vi "Drive Playback.vi"() -> ()   [LabVIEW 2010]
uses:
  <vilib>/NXT/Subs/MotorXNode.DC Motor Type.ctl
  <vilib>/NXT/Subs/LVHSConnector.ctl
  <vilib>/NXT/NXTIO Xnodes/NXTIOXNode/NXTIO.xnode
  <vilib>/NXT/Subs/MotorXNode.2DCMotor.ctl
  <vilib>/NXT/NXTIO Xnodes/AddressXNode/NXTIOAddress.xnode
  4150_RingItUp_State/4150_RingItUp_State.lvrbt
  <vilib>/NXT/NXTIO Xnodes/NXTIONodeSubVIs/TETRIX IO Move DC Motors.vi
panel:
  in  "DriveData":i8[][](array[numeric])
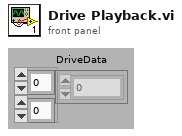
[diagram p1: front panel]
types:
  T1 = typedef "MotorXNode.DC Motor Type.ctl" = enum16{"DC Motor"}
  T2 = cluster{"DC Motor":T1, "Address":i16, "Address":i16}
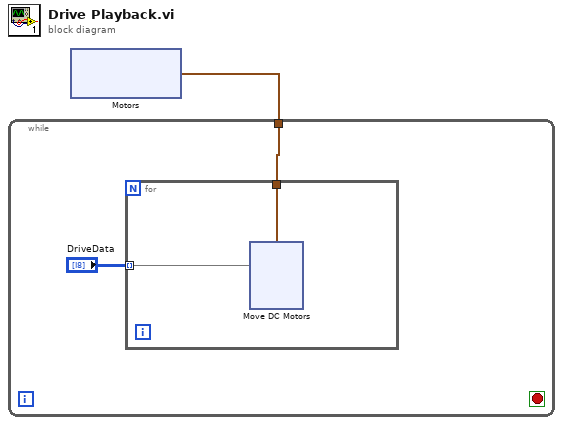
[diagram p0: block diagram]
diagram:
  n1 = xnode ("Motors")() -> ("DC Motor"=w1:T2)
  n2 = while {
    tunnel: w1 -> [w2]
    stop <- _ stop-if-true
    n3 = for {
      tunnel: "DriveData" -> [w5] mode=indexing
      tunnel: w2 -> [w4]
      n4 = xnode "Move DC Motors"("Power/Speed 1"=w5, "Motors"=w4) -> ()  [unwired: 2 in, 1 out]
    }
  }
